vi "IC_GPin.vi"(0 "ICImagingControl 3":refnum<k7>) -> (1 "ICImagingControl 2":refnum<k7>, 2 "GP In":i32)   [LabVIEW 2010]
doc: "Reads the state of the GP Input of a camera."
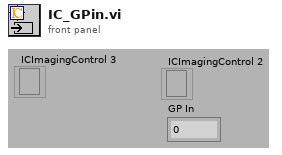
[diagram p1: front panel]
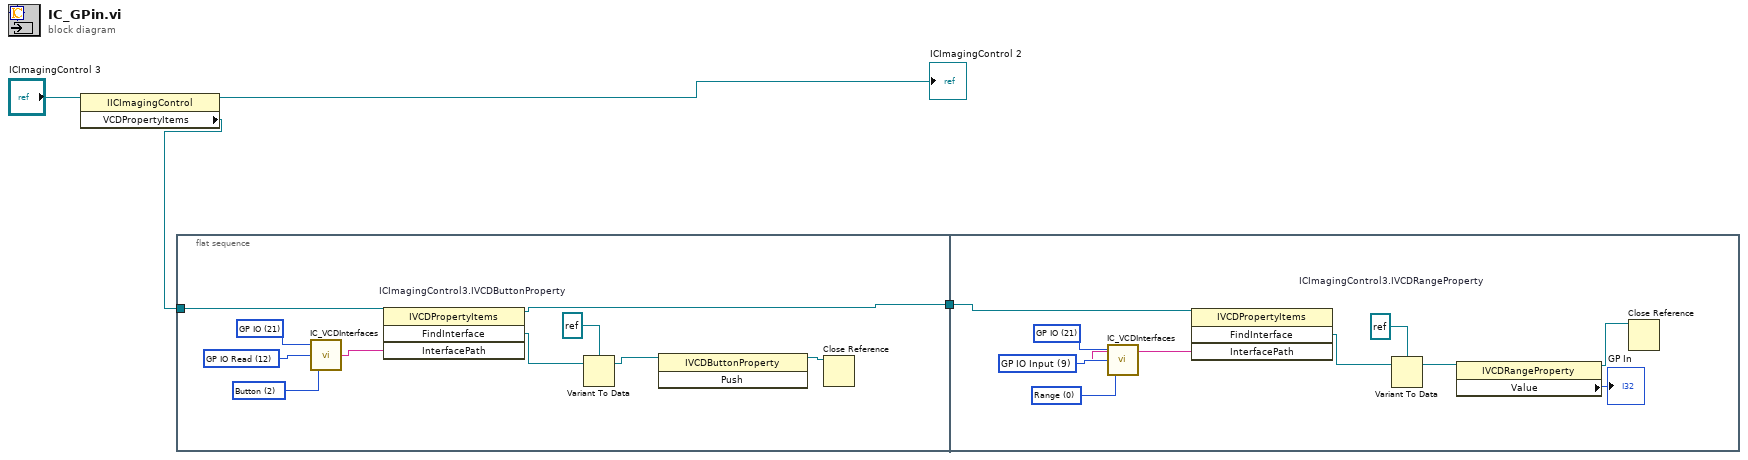
[diagram p0: block diagram]
diagram:
  n1 = property class="IICImagingControl"(reference="ICImagingControl 3") -> (reference out=→"ICImagingControl 2":refnum<k7>, "VCDPropertyItems"=w2:refnum<k7>)  [unwired: 1 in, 1 out]
  n2 = flat-sequence {
    tunnel: w2 -> [w10]
    tunnel: [w5] -> w1
    tunnel: w1 -> [w20]
    frame #0 {
      w7 = u16 2 items=["Range", "Switch", "Button", "Mapstrings", "Absolute Values"] ("Interface")
      w8 = u16 12 items=["Value", "Auto", "One Push", "Whitebalance Bue", "Whitebalance Red", "Auto Reference", "Trigger Polarity", "Trigger Mode", "Reset Value", "GP IO Input", "GP IO Output", "GP IO Write", "GP IO Read", "Strope Polarity", "Strobe Duration", "Strobe Delay"] ("Element ID")
      w9 = u16 21 items=["Brightness", "Contrast", "Hue", "Saturation", "Sharpness", "Gamma", "Color Enable", "White Balance", "Backlight Compensation", "Gain", "Pan", "Tilt", "Roll", "Zoom", "Exposure", "Iris", "Focus", "Trigger Mode", "VCR Compatibility", "Signal Detected", "Testpattern", "GP IO", "Strobe"] ("Property")
      w13 = refnum<k7> refnum  # ICImagingControl3.IVCDButtonProperty
      n3 = call <userlib>:"IC_VCDInterfaces.vi"("Interface"=w7, "Element ID"=w8, "Property"=w9) -> ("Interface Path"=w6:string)
      n4 = invoke class="IVCDPropertyItems" method="FindInterface"(reference=w10, "InterfacePath"=w6) -> (reference out=w5:refnum<k7>, "FindInterface"=w14:refnum<k7>)  [unwired: 2 in, 2 out]
      n5 = Variant To Data(Variant=w14, type=w13) -> (data=w12:refnum<k7>)  [unwired: 1 in, 1 out]
      n6 = invoke class="IVCDButtonProperty" method="Push"(reference=w12) -> (reference out=w11:refnum<k7>)  [unwired: 2 in, 2 out]
      n7 = Close Reference(reference=w11) -> ()  [unwired: 1 in, 1 out]
    }
    frame #1 {
      w17 = u16 0 items=["Range", "Switch", "Button", "Mapstrings", "Absolute Values"] ("Interface")
      w18 = u16 9 items=["Value", "Auto", "One Push", "Whitebalance Bue", "Whitebalance Red", "Auto Reference", "Trigger Polarity", "Trigger Mode", "Reset Value", "GP IO Input", "GP IO Output", "GP IO Write", "GP IO Read", "Strope Polarity", "Strobe Duration", "Strobe Delay"] ("Element ID")
      w19 = u16 21 items=["Brightness", "Contrast", "Hue", "Saturation", "Sharpness", "Gamma", "Color Enable", "White Balance", "Backlight Compensation", "Gain", "Pan", "Tilt", "Roll", "Zoom", "Exposure", "Iris", "Focus", "Trigger Mode", "VCR Compatibility", "Signal Detected", "Testpattern", "GP IO", "Strobe"] ("Property")
      w23 = refnum<k7> refnum  # ICImagingControl3.IVCDRangeProperty
      n8 = call <userlib>:"IC_VCDInterfaces.vi"("Interface"=w17, "Element ID"=w18, "Property"=w19) -> ("Interface Path"=w16:string)
      n9 = invoke class="IVCDPropertyItems" method="FindInterface"(reference=w20, "InterfacePath"=w16) -> ("FindInterface"=w24:refnum<k7>)  [unwired: 2 in, 3 out]
      n10 = Variant To Data(Variant=w24, type=w23) -> (data=w22:refnum<k7>)  [unwired: 1 in, 1 out]
      n11 = property class="IVCDRangeProperty"(reference=w22) -> (reference out=w21:refnum<k7>, "Value"=→"GP In":i32)  [unwired: 1 in, 1 out]
      n12 = Close Reference(reference=w21) -> ()  [unwired: 1 in, 1 out]
    }
  }
